vi "analoggingdata.vi"() -> ()   [LabVIEW 2018]
uses:
  <vilib>/Analysis/baseanly.llb/Mean (DBL).vi
  <vilib>/Analysis/NI_AALBase.lvlib
panel:
  in  "stop":bool
  out "min value":dbl
  out "max value":dbl
  out "mean":dbl
  out "current data point":dbl
  out "current data":dbl
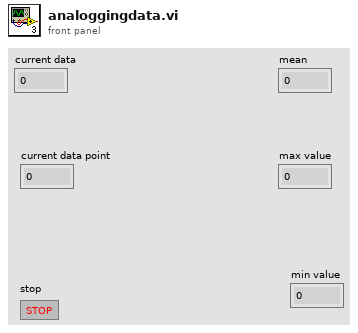
[diagram p1: front panel]
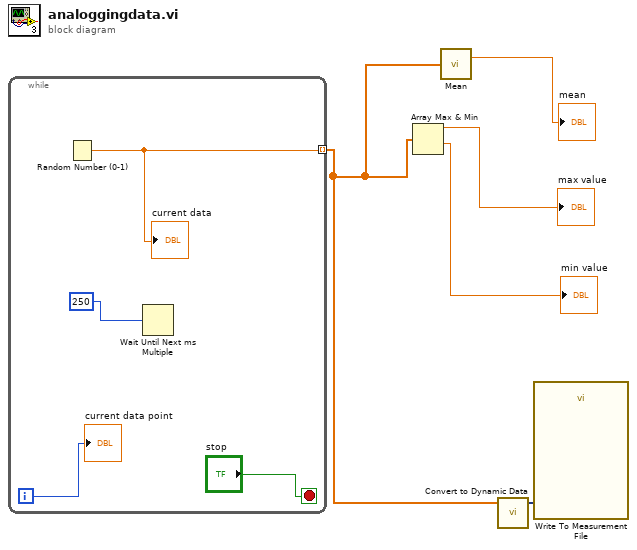
[diagram p0: block diagram]
diagram:
  n1 = while {
    tunnel: [w7] -> w1 mode=indexing
    i -> [w8]
    stop <- "stop" stop-if-true
    n2 = Random Number (0-1)() -> (number: 0 to 1=w7:dbl)
    "current data" <- w7
    n3 = Wait Until Next ms Multiple(millisecond multiple=250) -> ()  [unwired: 1 out]
    "current data point" <- w8
  }
  n4 = Array Max & Min(array=w1) -> (max value=→"max value":dbl, min value=→"min value":dbl)  [unwired: 2 out]
  n5 = call-poly <vilib>:"Mean.vi"("X"=w1) -> ("mean"=→"mean":dbl)  [unwired: 1 out]
  n6 = call "Convert to Dynamic Data"("Array"=w1) -> ("Dynamic Data Type"=w5:dynamicdata)  [unwired: 3 in]
  n7 = call "Write To Measurement File"("Signals"=w5) -> ()  [unwired: 16 in, 3 out]
